vi "DSF.Execution.Runtime.Plugin Manager.Query Disk for Plugin Classes.vi"(8 "error in (no error)":errorcluster, 9 "Plugin name":string, 10 "Plugins folder":path, 11 "Plugin Manager in":refnum<class "Plugin Manager.lvclass">) -> (0 "error out":errorcluster, 2 "Plugin class paths":path[](array[path]), 3 "Plugin Manager out":refnum<class "Plugin Manager.lvclass">)   [LabVIEW 2016, in "DSF.Engine.lvlib" / "Plugin Manager.lvclass"]
uses:
  Plugin Manager.lvclass
  <vilib>/Utility/libraryn.llb/Recursive File List.vi
  <vilib>/Utility/libraryn.llb/Check if File or Folder Exists.vi
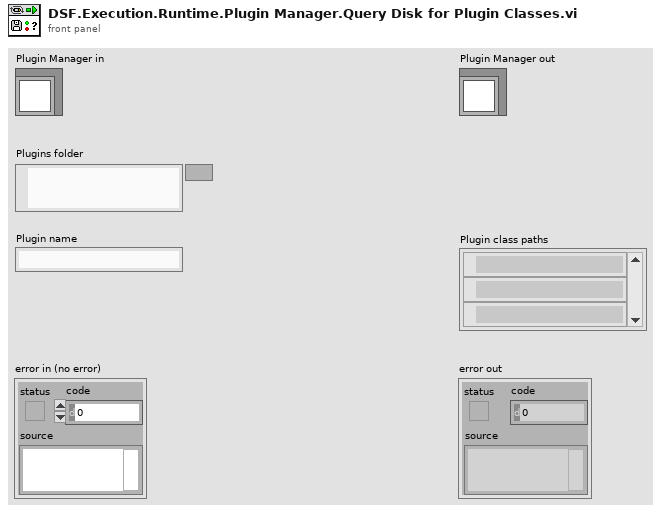
[diagram p1: front panel]
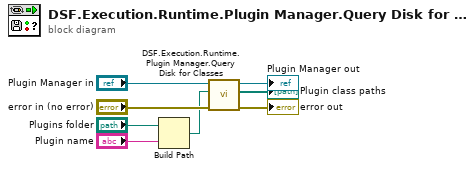
[diagram p0: block diagram]
diagram:
  n1 = Build Path(base path="Plugins folder", name or relative path="Plugin name") -> (appended path=w2:path)
  n2 = call "DSF.Execution.Runtime.Plugin Manager.Query Disk for Classes.vi"("error in (no error)"="error in (no error)", "folder"=w2, "Plugin Manager in"="Plugin Manager in") -> ("error out"=→"error out":errorcluster, "class paths"=→"Plugin class paths":path[], "Plugin Manager out"=→"Plugin Manager out":refnum<class "Plugin Manager.lvclass">)  [unwired: 6 in]
